vi "Spartan HTTP Verify Request Permission.vi"(11 "env":T1) -> (0 "reply":T3, 1 "process":bool, 2 "accessed document":string, 3 "env out":T1, 4 "script alias":bool, 5 "request type":T2=enum."CGI Movie")   [LabVIEW 2011]
uses:
  ITK EXT/http/cgi.llb/CGI Reply.ctl
  ITK EXT/utils/keyedarr.llb/Keyed Array.ctl
  ITK EXT/http/http1.llb/HTTP Request Type.ctl
  ITK EXT/http/config.llb/HTTP SRM.vi
panel:
  out "extension":string
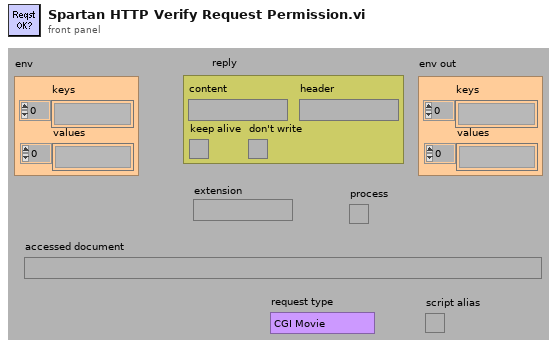
[diagram p1: front panel]
types:
  T1 = typedef "Keyed Array.ctl" = cluster{"keys":string[], "values":string[]}
  T2 = typedef "HTTP Request Type.ctl" = enum16{"Default", "Panel Picture", "Panel Movie", "CGI Movie"}
  T3 = typedef "CGI Reply.ctl" = cluster{"content":string, "header":string, "keep alive":bool, "don't write":bool}
  T4 = cluster{"value":string, "value":string, "value":string}
  T5 = cluster{cluster{"value":string, "value":string, "value":string}, cluster{"value":string, "value":string, "value":string}}
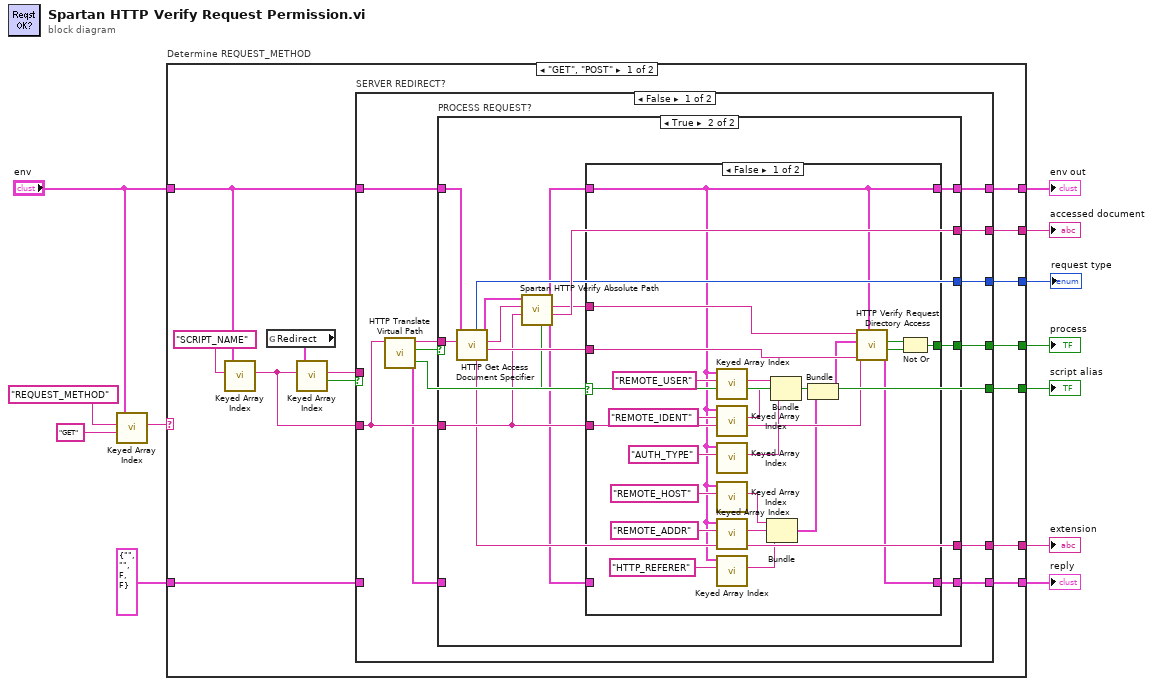
[diagram p0: block diagram]
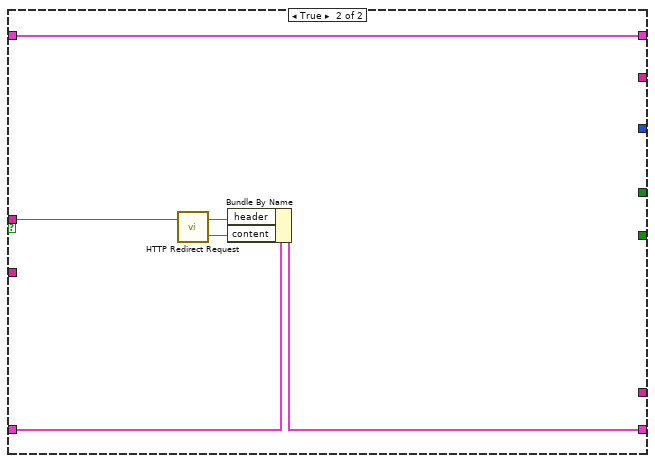
[diagram p4: hidden frame]
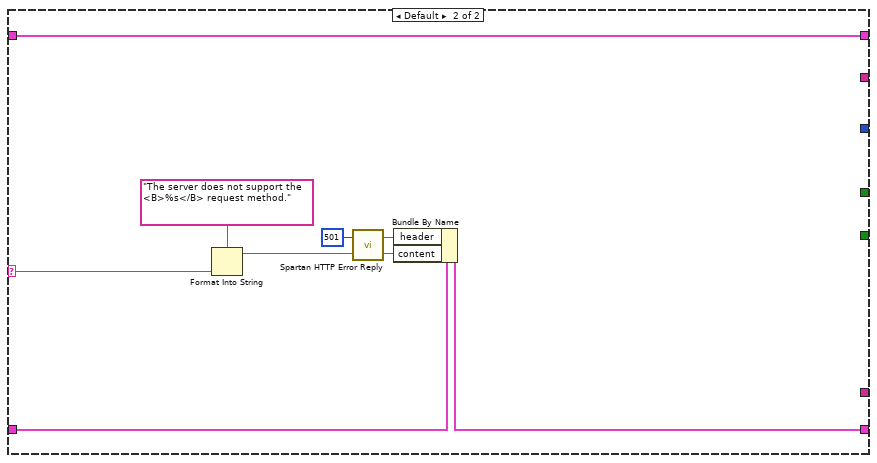
[diagram p5: hidden frame]
diagram:
  n1 = call "Keyed Array Index.vi"("default value"="GET", "key"="REQUEST_METHOD" ("name"), "array in"="env") -> ("value"=w8:string)  [unwired: 1 in, 3 out]
  n2 = case "Determine REQUEST_METHOD" shown="\"GET\", \"POST\"" w8 {
    selector: w8 -> [_ w90]
    tunnel: [w24 w95] -> w7
    tunnel: [w23 _] -> w12
    tunnel: [w22 w96] -> w6
    tunnel: "env" -> [w20 w96]
    tunnel: T3 {"content"="", "header"="", "keep alive"=FALSE, "don't write"=FALSE} ("Empty Reply") -> [w19 w88]
    tunnel: [w17 _] -> w4
    tunnel: [w16 _] -> w3
    tunnel: [w15 _] -> w2
    tunnel: [w14 _] -> w1
    frame "GET", "POST" {
      n3 = call "Keyed Array Index.vi"("key"="SCRIPT_NAME" ("name"), "array in"=w20) -> ("value"=w21:string)  [unwired: 2 in, 3 out]
      n4 = global read "HTTP SRM.vi" "Redirect"() -> (w13:T1)
      n5 = call "Keyed Array Index.vi"("key"=w21, "array in"=w13) -> ("valid key"=w26:bool, "value"=w25:string)  [unwired: 2 in, 2 out]
      n6 = case "SERVER REDIRECT?" shown="False" w26 {
        tunnel: w25 -> [_ w87]
        tunnel: w21 -> [w33 _]
        tunnel: [w38 w84] -> w24
        tunnel: [w37 _] -> w23
        tunnel: [w35 w83] -> w22
        tunnel: w20 -> [w34 w83]
        tunnel: w19 -> [_ w82]
        tunnel: [w31 _] -> w17
        tunnel: [w29 _] -> w16
        tunnel: [w28 _] -> w15
        tunnel: [w27 _] -> w14
        frame False {
          n7 = call "HTTP Translate Virtual Path.vi"("virtual path"=w33) -> ("reply"=w30:T3, "process"=w36:bool, "real path"=w32:string, "script alias"=w29:bool)  [unwired: 1 in, 6 out]
          n8 = case "PROCESS REQUEST?" shown="True" w36 {
            tunnel: w32 -> [_ w51]
            tunnel: [_ w56] -> w37
            tunnel: [w40 w55] -> w38
            tunnel: w30 -> [w40 _]
            tunnel: w33 -> [_ w53]
            tunnel: [w39 w50] -> w35
            tunnel: w34 -> [w39 w52]
            tunnel: [_ w48] -> w31
            tunnel: [_ w46] -> w28
            tunnel: [_ w45] -> w27
            frame False {
            }
            frame True {
              n9 = call "HTTP Get Access Document Specifier.vi"("absolute path"=w51, "env"=w52) -> ("method"=w54:string, "accessed document"=w49:string, "env out"=w47:T1, "extension"=w45:string, "request type"=w46:T2)  [unwired: 5 out]
              n10 = call "Spartan HTTP Verify Absolute Path.vi"("request"=w53, "absolute path"=w49, "env"=w47) -> ("reply"=w43:T3, "document path"=w48:string, "document directory path"=w42:string, "env out"=w41:T1, "failed"=w44:bool)  [unwired: 1 in, 3 out]
              n11 = case shown="False" w44 {
                tunnel: w54 -> [w74 _]
                tunnel: w53 -> [w75 _]
                tunnel: [w79 w81] -> w55
                tunnel: [w77 _] -> w56
                tunnel: w43 -> [_ w81]
                tunnel: w42 -> [w73 _]
                tunnel: w41 -> [w58 w80]
                tunnel: [w58 w80] -> w50
                frame False {
                  n12 = call "Keyed Array Index.vi"("key"="REMOTE_USER", "array in"=w58) -> ("value"=w66:string)  [unwired: 2 in, 3 out]
                  n13 = call "Keyed Array Index.vi"("key"="REMOTE_IDENT", "array in"=w58) -> ("value"=w67:string)  [unwired: 2 in, 3 out]
                  n14 = call "Keyed Array Index.vi"("key"="AUTH_TYPE", "array in"=w58) -> ("value"=w68:string)  [unwired: 2 in, 3 out]
                  n15 = call "Keyed Array Index.vi"("key"="REMOTE_HOST", "array in"=w58) -> ("value"=w64:string)  [unwired: 2 in, 3 out]
                  n16 = call "Keyed Array Index.vi"("key"="REMOTE_ADDR", "array in"=w58) -> ("value"=w63:string)  [unwired: 2 in, 3 out]
                  n17 = call "Keyed Array Index.vi"("key"="HTTP_REFERER", "array in"=w58) -> ("value"=w62:string)  [unwired: 2 in, 3 out]
                  n18 = Bundle("value"=w64, "value"=w63, "value"=w62) -> (w72:T4)  [unwired: 1 out]
                  n19 = Bundle("value"=w66, "value"=w67, "value"=w68) -> (w65:T4)  [unwired: 1 out]
                  n20 = Bundle(w65, w72) -> (w57:T5)  [unwired: 1 out]
                  n21 = call "HTTP Verify Request Directory Access.vi"("env"=w58, "method"=w74, "request"=w75, "access info"=w57, "absolute path"=w73) -> ("reply"=w79:T3, "failed"=w76:bool, "auth required"=w78:bool)  [unwired: 4 out]
                  n22 = Not Or(1:w76, 2:w78) -> (0:w77:bool)
                }
                frame True {
                }
              }
            }
          }
        }
        frame True {
          n23 = call "HTTP Redirect Request.vi"("new location"=w87) -> ("content"=w85:string, "header"=w86:string)  [unwired: 1 out]
          n24 = Bundle By Name(cluster=w82, "header"=w86, "content"=w85) -> (w84:T3)
        }
      }
    }
    frame Default {
      n25 = Format Into String(format string="The server does not support the <B>%s</B> request method.", w90) -> (resulting string=w89:string)  [unwired: 2 in, 1 out]
      n26 = call "Spartan HTTP Error Reply.vi"("message"=w89, "status code"=501) -> ("content"=w93:string, "header"=w94:string)
      n27 = Bundle By Name(cluster=w88, "header"=w94, "content"=w93) -> (w95:T3)
    }
  }
  "reply" <- w7
  "process" <- w12
  "env out" <- w6
  "accessed document" <- w4
  "script alias" <- w3
  "request type" <- w2
  "extension" <- w1
